vi "Read Handle.vi"(8 "error in":errorcluster, 11 "Configurable Device in":refnum<class "Configurable Device.lvclass">) -> (0 "error out":errorcluster, 2 "Config Data Session Out":refnum<data-value>, 3 "Configurable Device out":refnum<class "Configurable Device.lvclass">)   [LabVIEW 2017, in "Configurable Device.lvclass"]
uses:
  Configurable Device.lvclass
  <vilib>/MSR Consulting, LLC/General Reuse/Session APIs/File Access/Config Data/Config Data.lvclass
  Configurable Device.lvclass/Configurable Device.ctl
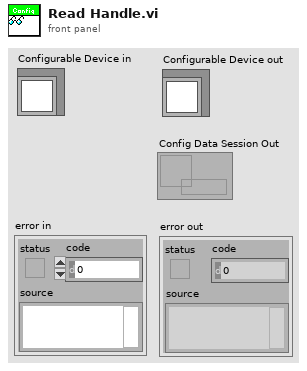
[diagram p1: front panel]
types:
  T1 = typedef "Session - Root.lvclass/Session Handle.ctl" = refnum<data-value>
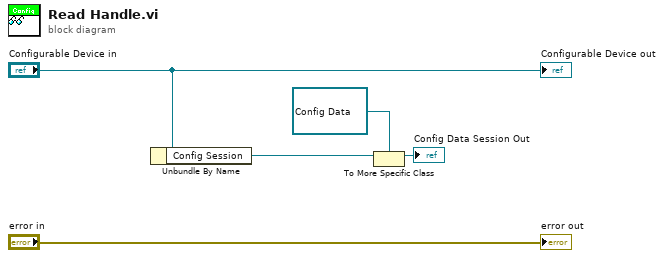
[diagram p0: block diagram]
diagram:
  n1 = Unbundle By Name("Configurable Device in") -> ("Config Session"=w3:T1)
  n2 = To More Specific Class(target class=refnum<data-value> refnum, reference=w3) -> (specific class reference=→"Config Data Session Out":refnum<data-value>)  [unwired: 1 in, 1 out]
  "error out" <- "error in"
  "Configurable Device out" <- "Configurable Device in"
